vi "Get DAC Offset_CK.vi"(4 "error in (no error)":errorcluster, 5 "Wait before read (0ms)":u32=10, 6 "Axis (1)":i32=1 min=1 max=3, 7 "VISA resource name":refnum<visa-resource-name>) -> (0 "error out":errorcluster, 2 "DAC Offset":dbl format="%.6g", 3 "VISA resource name out":refnum<visa-resource-name>)   [LabVIEW 2013]
doc: "Returns the DAC offset value."
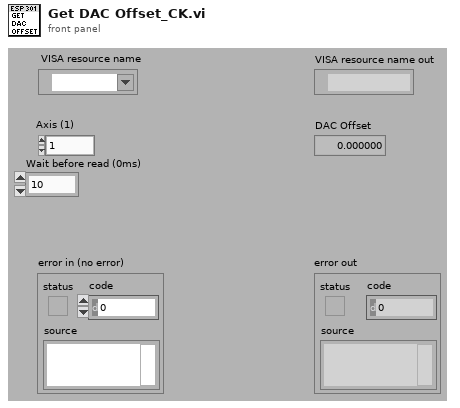
[diagram p1: front panel]
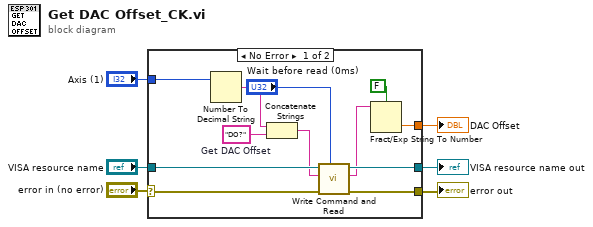
[diagram p0: block diagram]
diagram:
  n1 = case shown="No Error" "error in (no error)" {
    selector: "error in (no error)" -> [w15 w20]
    tunnel: [w17 w20] -> w6
    tunnel: "VISA resource name" -> [w18 w19]
    tunnel: [w16 w19] -> w5
    tunnel: [w13 _] -> w2
    tunnel: "Axis (1)" -> [w10 _]
    frame No Error {
      w12 = "DO?"  # Get DAC Offset
      n2 = Number To Decimal String(number=w10) -> (decimal integer string=w11:string)  [unwired: 1 out]
      n3 = Concatenate Strings(w11, w12) -> (w9:string)
      n4 = call <instrlib>:"Write Command and Read.vi"("Wait before read (0ms)"="Wait before read (0ms)", "error in (no error)"=w15, "Command"=w9, "VISA resource name"=w18) -> ("error out"=w17:errorcluster, "Returned string"=w14:string, "VISA resource name out"=w16:refnum<visa-resource-name>)  [unwired: 1 in, 2 out]
      n5 = Fract/Exp String To Number(use system decimal point (T)=FALSE ("utiliser le séparateur décimal du système (V)"), string=w14) -> (number=w13:dbl)  [unwired: 3 out]
    }
    frame Error {
    }
  }
  "error out" <- w6
  "VISA resource name out" <- w5
  "DAC Offset" <- w2
